vi "EnvCoverGetState.vi"(8 "error in (no error)":errorcluster) -> (0 "error out":errorcluster, 3 "MotorState Out":T1)   [LabVIEW 2016]
uses:
  controls/MotorStates.ctl
  controls/RT-Variables.lvlib
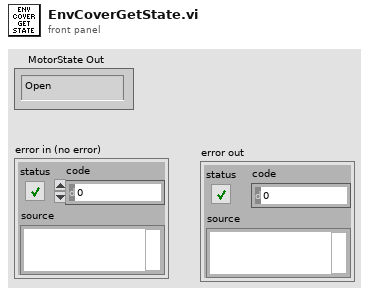
[diagram p1: front panel]
types:
  T1 = typedef "RT-Variables.lvlib/MotorStates.ctl" = enum16{"Open", "Close", "Moving", "Screwed"}
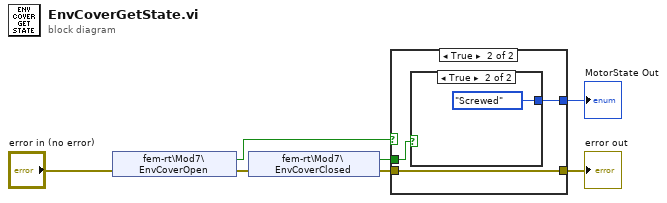
[diagram p0: block diagram]
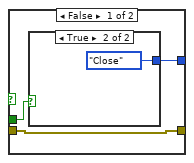
[diagram p2: hidden frame]
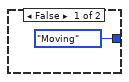
[diagram p3: hidden frame]
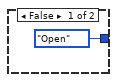
[diagram p4: hidden frame]
diagram:
  n1 = shared-variable "fem-rt\\Mod7\\EnvCoverOpen"(error in="error in (no error)") -> (w7:bool, error out=w3:errorcluster)
  n2 = shared-variable "fem-rt\\Mod7\\EnvCoverClosed"(error in=w3) -> (w1:bool, error out=w2:errorcluster)
  n3 = case shown="True" w7 {
    tunnel: w2 -> [w9 w15]
    tunnel: [w9 w15] -> w4
    tunnel: [w10 w13] -> w5
    tunnel: w1 -> [w8 w14]
    frame False {
      n4 = case shown="True" w8 {
        tunnel: [MotorStates."Moving" ("MotorState") MotorStates."Close" ("MotorState")] -> w10
        frame False {
        }
        frame True {
        }
      }
    }
    frame True {
      n5 = case shown="True" w14 {
        tunnel: [MotorStates."Open" ("MotorState") MotorStates."Screwed" ("MotorState")] -> w13
        frame False {
        }
        frame True {
        }
      }
    }
  }
  "error out" <- w4
  "MotorState Out" <- w5
